vi "Write ElectrometerInternalConfiguration.lvclass.vi"(8 "error in (no error)":errorcluster, 10 "ElectrometerInternalConfiguration.lvclass":refnum<class "ElectrometerInternalConfiguration.lvclass">, 11 "Electrometer in":refnum<class "Electrometer.lvclass">) -> (0 "error out":errorcluster, 3 "Electrometer out":refnum<class "Electrometer.lvclass">)   [LabVIEW 2016, in "Electrometer.lvclass"]
uses:
  Electrometer.lvclass
  ElectrometerConfiguration/ElectrometerInternalConfiguration.lvclass
  Electrometer.lvclass/Electrometer.ctl
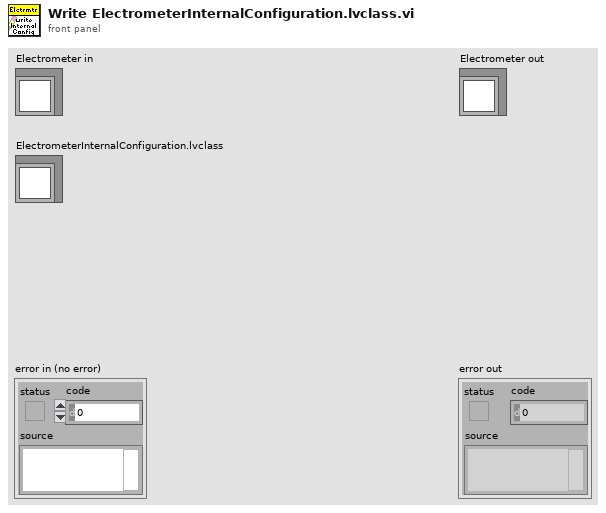
[diagram p1: front panel]
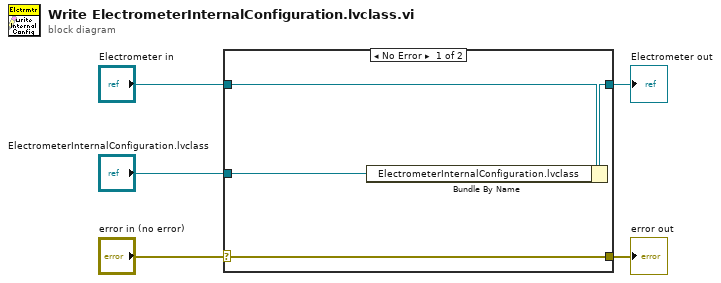
[diagram p0: block diagram]
diagram:
  n1 = case shown="No Error" "error in (no error)" {
    selector: "error in (no error)" -> [w9 w10]
    tunnel: [w9 w10] -> w4
    tunnel: [w7 w11] -> w2
    tunnel: "Electrometer in" -> [w8 w11]
    tunnel: "ElectrometerInternalConfiguration.lvclass" -> [w6 _]
    frame No Error {
      n2 = Bundle By Name(cluster=w8, "ElectrometerInternalConfiguration.lvclass"=w6) -> (w7:refnum<class "Electrometer.lvclass">)
    }
    frame Error {
    }
  }
  "error out" <- w4
  "Electrometer out" <- w2
